vi "Disconnect from Slave.vi"(8 "error in (no error)":errorcluster, 11 "network master in":refnum<class "WebSocket Client CR.lvclass">) -> (0 "error out":errorcluster, 3 "network master out":refnum<class "WebSocket Client CR.lvclass">)   [LabVIEW 2021, in "WebSockets.lvlib" / "WebSocket Client CR.lvclass"]
doc: "This provides an interface for the master to open a connection to the slave."
uses:
  WebSocket Client CR.lvclass
  WebSocket Client CR.lvclass/WebSocket Client CR.ctl
  WebSocket/WebSocket.lvclass
  Sockets/Socket/Socket.lvclass
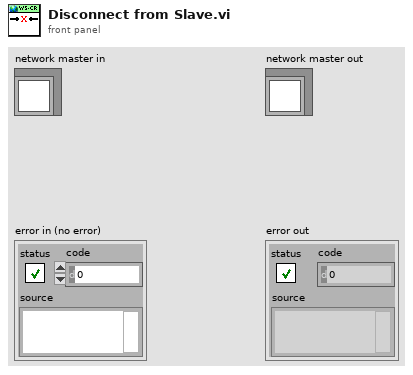
[diagram p1: front panel]
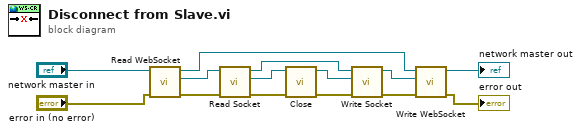
[diagram p0: block diagram]
diagram:
  n1 = call "Read WebSocket.vi"("error in (no error)"="error in (no error)", "Master CR in"="network master in") -> ("error out"=w13:errorcluster, "WebSocket"=w14:refnum<class "WebSocket.lvclass">, "Master CR out"=w9:refnum<class "WebSocket Client CR.lvclass">)  [unwired: 7 in]
  n2 = call "Read Socket.vi"("error in (no error)"=w13, "WebSocket in"=w14) -> ("error out"=w6:errorcluster, "Socket"=w4:refnum<class "Socket.lvclass">, "WebSocket out"=w10:refnum<class "WebSocket.lvclass">)  [unwired: 7 in]
  n3 = call-dynamic "Close.vi"("error in (no error)"=w6, "Socket in"=w4) -> ("error out"=w5:errorcluster, "Socket out"=w3:refnum<class "Socket.lvclass">)  [unwired: 8 in]
  n4 = call "Write Socket.vi"("error in (no error)"=w5, "Socket"=w3, "WebSocket in"=w10) -> ("error out"=w12:errorcluster, "WebSocket out"=w11:refnum<class "WebSocket.lvclass">)  [unwired: 7 in]
  n5 = call "Write WebSocket.vi"("error in (no error)"=w12, "WebSocket"=w11, "Master CR in"=w9) -> ("error out"=→"error out":errorcluster, "Master CR out"=→"network master out":refnum<class "WebSocket Client CR.lvclass">)  [unwired: 7 in]
